vi "Display Three Button Popup (Plain).vi"(5 "Action 1 Text":string="No", 6 "Theme":refnum<class "Theme.lvclass">, 7 "Action 0 Text":string="Yes", 8 "error in":errorcluster, 9 "Action 2 Text":string="No", 10 "Message":string, 11 "Dialog Title":string) -> (0 "error out":errorcluster, 1 "Choice":u8)   [LabVIEW 2021, in "Pop-Up.lvlib" / "Plain - Three Button.lvclass"]
doc: "The one button popup will display information to the user and wait for the operator to click the button.\n\n<b>Note:</b> The function <b>Close Pop-Up.vi</b> can be used to close this dialog early.\n\n<b>Note:</b> The dialog vertical sizing will adjust for longer messages, so <b>test</b> all messages prior to deployment to make sure that scaling fits.\n\nInputs:\n-Dialog Title [String] - String variable to populate the dialog's title bar\n-Message [String] - String Variable to populate Display\n-Theme [lvclass] - the theme for the style of the popup\n-Action 0 [String] - the button text for the <b>Action 0</b> button (far right)\n-Action 1 [String] - the button text for the <b>Action 1</b> button (middle)\n-Action 2 [String] - the button text for the <b>Action 2</b> button (far left)\n\nOutputs:\n-Choice [U8] - user selection of button 0, 1, or 2\n\n<b>Code Developed By:</b>\nDaniel Coons\nTechnology Service Corporation\n1983 S Liberty Drive\nBloomington, IN 47403\nPhone: 812 558-7100\ndaniel.coons@tsc.com\nwww.tsc.com/atcs"
uses:
  Plain - Three Button.lvclass
  Theme/Theme.lvclass
  C:/Development/Open Source/tsc-pop-up/Popup/Popup.lvclass
  C:/Development/Open Source/tsc-pop-up/Plain/Plain Parent.lvclass
  Plain Parent.lvclass/Plain Parent.ctl
  Plain - Three Button.lvclass/Plain - Three Button.ctl
  Write Dialog Title.vi
  Write Action 1 Text.vi
  Write Action 2 Text.vi
  Write Action 3 Text.vi
  Popup/Data Member Access/Write Theme.vi
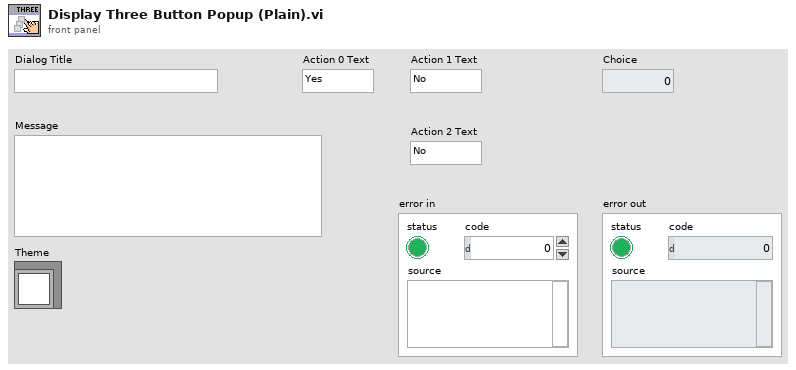
[diagram p1: front panel]
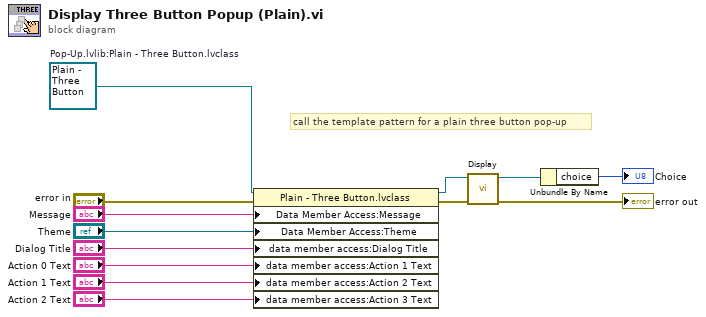
[diagram p0: block diagram]
diagram:
  w1 = refnum<class "Plain - Three Button.lvclass"> refnum  # Pop-Up.lvlib:Plain - Three Button.lvclass
  # "call the template pattern for a plain three button pop-up"
  n1 = property class="Plain - Three Button.lvclass"(reference=w1, error in="error in", "Data Member Access:Message"="Message", "Data Member Access:Theme"="Theme", "data member access:Dialog Title"="Dialog Title", "data member access:Action 1 Text"="Action 0 Text", "data member access:Action 2 Text"="Action 1 Text", "data member access:Action 3 Text"="Action 2 Text") -> (reference out=w10:refnum<class "Plain - Three Button.lvclass">, error out=w11:errorcluster)
  n2 = call-dynamic "Display.vi"("error in"=w11, "Plain - Three Button in"=w10) -> ("error out"=→"error out":errorcluster, "Plain - Three Button out"=w3:refnum<class "Plain - Three Button.lvclass">)  [unwired: 8 in]
  n3 = Unbundle By Name(w3) -> ("choice"=→"Choice":u8)
